vi "TwoColorSensor.vi"   [LabVIEW 2016, in "TestColorSensor.lvrbt"]
uses:
  TestColorSensor.lvrbt
  <vilib>/NXT/Block Support/NXT_InputPort.ctl
  <vilib>/NXT/Dual Mode Library/Sensors/Light_On.vi
  <vilib>/NXT/Dual Mode Library/Display/drawNumber_float.vi
types:
  T1 = typedef "NXT_InputPort.ctl" = u32
  T2 = typedef "LVHSConnector.ctl" = refnum<class "BrickReference.lvclass">
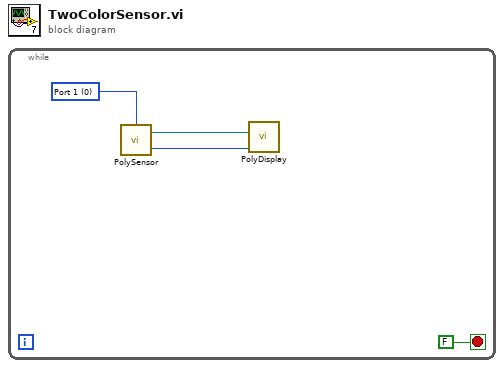
[diagram p0: block diagram]
diagram:
  n1 = while {
    stop <- FALSE stop-if-true
    w4 = T1 0 items=["Port 1", "Port 2", "Port 3", "Port 4"] ("Port (Port 1)")
    n2 = call-poly <vilib>:"PolySensor.vi"("Port (Port 3)"=w4) -> ("Scaled Value"=w1:i16, "NXT/EV3"=w2:T2)  [unwired: 2 in]
    n3 = call-poly <vilib>:"PolyDisplay.vi"("number"=w1, "NXT/EV3"=w2) -> ()  [unwired: 2 in, 1 out]
  }
